vi "Directional Speed Sensors Page.vi"(8 "error in (no error)":errorcluster, 11 "Node Ptr":T1 format="%.0x") -> (0 "error out":errorcluster)   [LabVIEW 2013, in "Engine Simulation Toolkit System Explorer.lvlib"]
uses:
  Engine Simulation Toolkit System Explorer.lvlib
  <vilib>/NI Veristand/Custom Device API/Custom Device Item Ref.ctl
  Shared/Properties.vi
  Shared/Constants and GUIDs.vi
  <vilib>/NI Veristand/Custom Device API/Custom Device API.lvlib
  Shared/Engine Simulation Toolkit Shared.lvlib
  <vilib>/NI Veristand/Custom Device Tools/Custom Device Utility Library/Custom Device Utility Library.lvlib
panel:
  in  "remove":bool
  in  "add":bool
  in  "DirSpeed listbox":i32[](listbox) caption="Available Directional Speed Sensors"
  in  "Header":cluster{"Section Name":string}={"Section Name"="Directional Speed Sensors"}
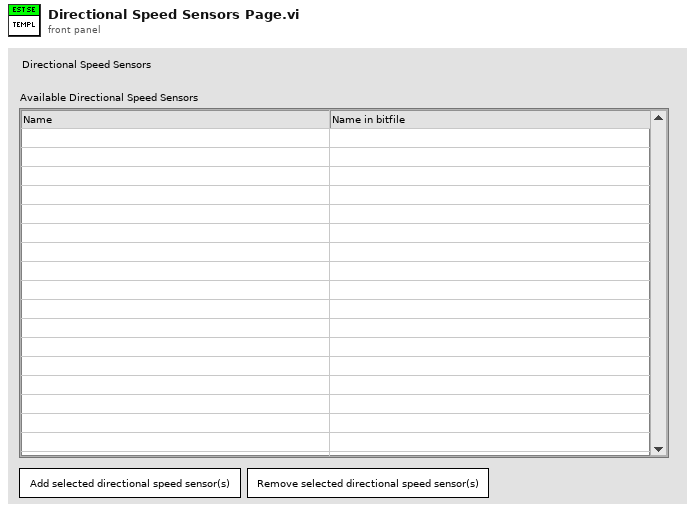
[diagram p1: front panel]
types:
  T1 = typedef "Custom Device API.lvlib/Custom Device Item Ref.ctl" = u64
  T2 = enum8{"Enabled", "Disabled", "Disabled and Grayed Out"}
  T3 = typedef "Custom Device API.lvlib/Custom Device Commands.ctl" = enum16{"Default", "Item renamed", "Shutdown", "Dynamic button pressed"}
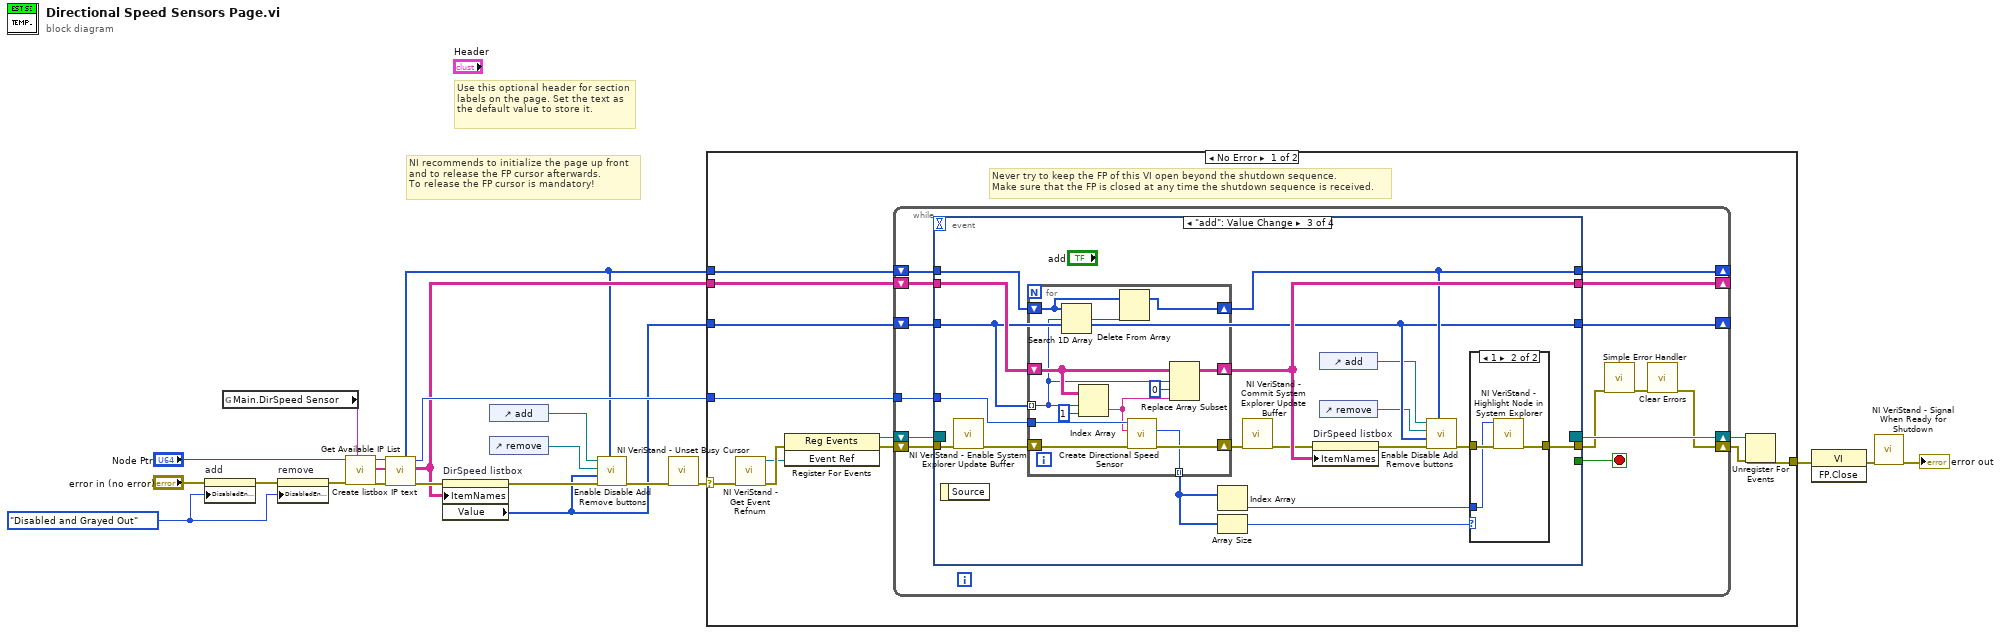
[diagram p0: block diagram]
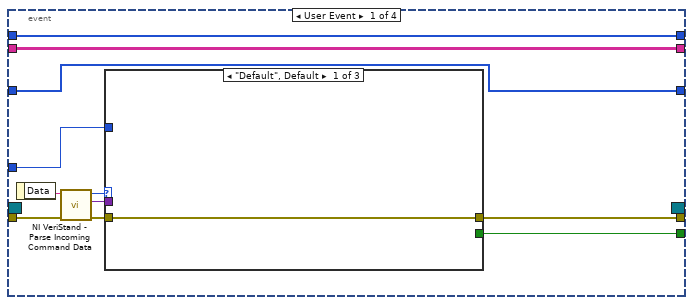
[diagram p2: hidden frame]
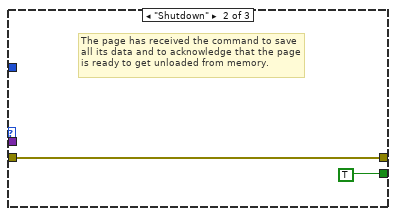
[diagram p3: hidden frame]
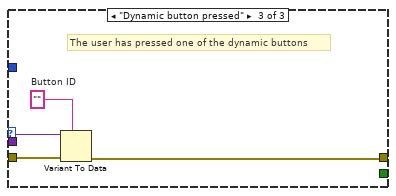
[diagram p4: hidden frame]
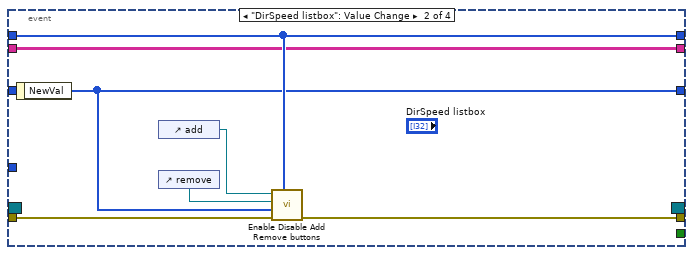
[diagram p5: hidden frame]
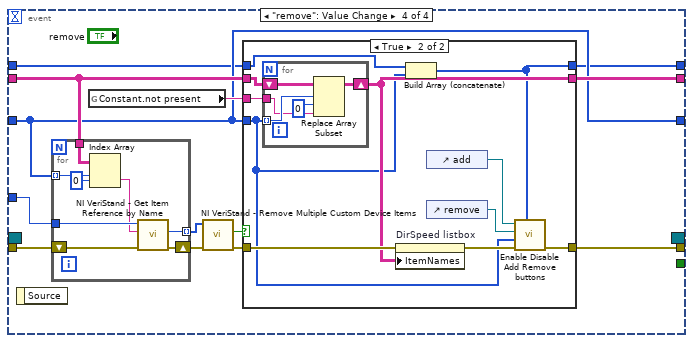
[diagram p7: hidden frame]
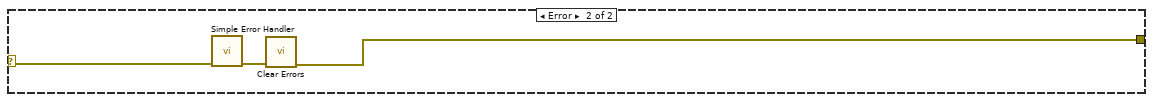
[diagram p9: hidden frame]
diagram:
  w7 = T2."Disabled and Grayed Out" ("Disabled")
  # "Use this optional header for section labels on the page. Set the text as the default value to store it."
  # "NI recommends to initialize the page up front\nand to release the FP cursor afterwards.\nTo release the FP cursor is mandatory!"
  n1 = property on="add" class="Bool"(error in="error in (no error)", "DisabledEnum"=w7) -> (error out=w9:errorcluster)  [unwired: 1 in, 1 out]
  n2 = global read "Properties.vi" "Main.DirSpeed Sensor"() -> (w15:string)
  n3 = property on="remove" class="Bool"(error in=w9, "DisabledEnum"=w7) -> (error out=w8:errorcluster)  [unwired: 1 in, 1 out]
  n4 = call "Get Available IP List.vi"("ip list property name"=w15, "error in (no error)"=w8, "Item Ref in"="Node Ptr") -> ("error out"=w17:errorcluster, "ips available"=w12:string[], "Item Ref out"=w14:T1)  [unwired: 6 in]
  n5 = call "Create listbox IP text.vi"("error in (no error)"=w17, "ips available"=w12, "Section Ref in"=w14) -> ("error out"=w11:errorcluster, "listbox text"=w10:string[][], "Section Ref out"=w13:T1, "not present item indexes"=w2:i32[])  [unwired: 5 in]
  n6 = property on="DirSpeed listbox" class="MCListbox (strict)"(error in=w11, "ItemNames"=w10) -> (error out=w4:errorcluster, "Value"=w1:i32[])  [unwired: 1 in, 1 out]
  n7 = control-ref of="add"() -> (w5:refnum<vi>)
  n8 = control-ref of="remove"() -> (w6:refnum<vi>)
  n9 = call "Enable Disable Add Remove buttons.vi"("not present item indexes"=w2, "error in (no error)"=w4, "selected items"=w1, "remove button"=w6, "add button"=w5) -> ("error out"=w3:errorcluster)  [unwired: 6 in]
  n10 = call <vilib>:"NI VeriStand - Unset Busy Cursor.vi"("error in (no error)"=w3) -> ("error out"=w19:errorcluster)  [unwired: 10 out]
  n11 = case shown="No Error" w19 {
    selector: w19 -> [w26 w151]
    tunnel: [w31 w149] -> w22
    tunnel: w13 -> [w27 _]
    tunnel: w10 -> [w25 _]
    tunnel: w2 -> [w24 _]
    tunnel: w1 -> [w23 _]
    frame No Error {
      # "Never try to keep the FP of this VI open beyond the shutdown sequence.\nMake sure that the FP is closed at any time the shutdown sequence is received."
      n12 = call <vilib>:"NI VeriStand - Get Event Refnum.vi"("error in (no error)"=w26) -> ("error out"=w34:errorcluster, "Event Ref"=w30:refnum<user-event>)  [unwired: 9 out]
      n13 = register-events(error in=w34, w30) -> (reference out=w28:refnum<event-registration>, error out=w29:errorcluster)  [unwired: 1 in]
      n14 = while {
        tunnel: w27 -> [w44]
        shift-right: [w41] -> w32
        shift-left: w29 -> [w47]
        shift-right: [w48] -> w33
        shift-left: w28 -> [w46]
        shift-right: [w38] -> _
        shift-left: w23 -> [w37]
        shift-right: [w35] -> _
        shift-left: w24 -> [w39]
        shift-right: [w36] -> _
        shift-left: w25 -> [w40]
        stop <- w45 stop-if-true
        n15 = event shown="[2] \"add\": Value Change" {
          selector: w46 -> [_ _ _ _]
          dyn-events: [_ _ _ _] -> w48
          timeout: _ -> [_ _ _ _]
          tunnel: w47 -> [w59 w73 w91 w120]
          tunnel: [w55 _ _ _] -> w45
          tunnel: [w54 w72 w76 w121] -> w43
          tunnel: w44 -> [w53 _ w90 w119]
          tunnel: w40 -> [w50 w67 w89 w114]
          tunnel: w39 -> [w49 w69 w88 w110]
          tunnel: [w51 w68 w83 w111] -> w38
          tunnel: w37 -> [w51 _ w83 w111]
          tunnel: [w50 w67 w86 w112] -> w36
          tunnel: [w49 w69 w84 w109] -> w35
          event User Event {
            n16 = event-data() -> ("Data"=w58:string)  [unwired: 1 out]
            n17 = call <vilib>:"NI VeriStand - Parse Incoming Command Data.vi"("error in (no error)"=w59, "Incoming data"=w58) -> ("error out"=w57:errorcluster, "Outgoing data"=w52:variant, "Action"=w56:T3)  [unwired: 7 out]
            n18 = case shown="\"Default\", Default" w56 {
              tunnel: w57 -> [w60 w61 w66]
              tunnel: [_ TRUE _] -> w55
              tunnel: [w60 w61 w63] -> w54
              tunnel: w53 -> [_ _ _]
              tunnel: w52 -> [_ _ w65]
              frame "Default", Default {
              }
              frame "Shutdown" {
                # "The page has received the command to save all its data and to acknowledge that the page is ready to get unloaded from memory."
              }
              frame "Dynamic button pressed" {
                w64 = ""  # Button ID
                # "The user has pressed one of the dynamic buttons"
                n19 = Variant To Data(error in=w66, type=w64, Variant=w65) -> (error out=w63:errorcluster)  [unwired: 1 out]
              }
            }
          }
          event "DirSpeed listbox": Value Change {
            n20 = event-data() -> ("NewVal"=w68:i32[])  [unwired: 1 out]
            n21 = control-ref of="add"() -> (w71:refnum<vi>)
            n22 = control-ref of="remove"() -> (w70:refnum<vi>)
            n23 = call "Enable Disable Add Remove buttons.vi"("not present item indexes"=w69, "error in (no error)"=w73, "selected items"=w68, "remove button"=w70, "add button"=w71) -> ("error out"=w72:errorcluster)  [unwired: 6 in]
          }
          event "add": Value Change {
            n24 = event-data() -> ()  [unwired: 2 out]
            n25 = call <vilib>:"NI VeriStand - Enable System Explorer Update Buffer.vi"("error in (no error)"=w91) -> ("error out"=w79:errorcluster)  [unwired: 10 in]
            n26 = for {
              tunnel: w90 -> [w106]
              shift-right: [w107] -> w87
              shift-left: w79 -> [w108]
              tunnel: w83 -> [w100] mode=indexing
              shift-right: [w103] -> w86
              shift-left: w89 -> [w104]
              shift-right: [w97] -> w84
              shift-left: w88 -> [w99]
              tunnel: [w96] -> w78 mode=indexing
              n27 = Search 1D Array(1D array=w99, element=w100) -> (index of element=w98:i32)  [unwired: 1 in]
              n28 = Index Array(array=w104, index (row)=w100, index (col)=1 ("disabled index (col)")) -> (element=w101:string)
              n29 = Delete From Array(array=w99, index=w98) -> (array with subset deleted=w97:i32[])  [unwired: 1 in, 1 out]
              n30 = call "Create Directional Speed Sensor.vi"("error in (no error)"=w108, "dir speed sensor name"=w101, "Section Ptr"=w106) -> ("error out"=w107:errorcluster, "dir speed sensor ref"=w96:T1)  [unwired: 6 in, 1 out]
              n31 = Replace Array Subset(array=w104, new element=w101, index (row)=w100, index (col)=0 ("disabled index (col)")) -> (w103:string[][])
            }
            n32 = Index Array(array=w78) -> (element=w74:T1)  [unwired: 1 in]
            n33 = Array Size(array=w78) -> (size(s)=w77:i32)
            n34 = call <vilib>:"NI VeriStand - Commit System Explorer Update Buffer.vi"("error in (no error)"=w87) -> ("error out"=w80:errorcluster)  [unwired: 10 in]
            n35 = property on="DirSpeed listbox" class="MCListbox (strict)"(error in=w80, "ItemNames"=w86) -> (error out=w85:errorcluster)  [unwired: 1 in, 1 out]
            n36 = control-ref of="add"() -> (w82:refnum<vi>)
            n37 = control-ref of="remove"() -> (w81:refnum<vi>)
            n38 = call "Enable Disable Add Remove buttons.vi"("not present item indexes"=w84, "error in (no error)"=w85, "selected items"=w83, "remove button"=w81, "add button"=w82) -> ("error out"=w75:errorcluster)  [unwired: 6 in]
            n39 = case shown="1" w77 {
              tunnel: [w92 w94] -> w76
              tunnel: w75 -> [w92 w95]
              tunnel: w74 -> [_ w93]
              frame Default {
              }
              frame 1 {
                n40 = call <vilib>:"NI VeriStand - Highlight Node in System Explorer.vi"("error in (no error)"=w95, "Item Ref in"=w93) -> ("error out"=w94:errorcluster)  [unwired: 8 in, 1 out]
              }
            }
          }
          event "remove": Value Change {
            n41 = event-data() -> ()  [unwired: 2 out]
            n42 = for {
              tunnel: w111 -> [w147] mode=indexing
              tunnel: w114 -> [w148]
              tunnel: w119 -> [w144]
              tunnel: [w141] -> w117 mode=indexing
              shift-right: [w143] -> w118
              shift-left: w120 -> [w145]
              n43 = Index Array(array=w148, index (row)=w147, index (col)=0 ("disabled index (col)")) -> (element=w142:string)
              n44 = call <vilib>:"NI VeriStand - Get Item Reference by Name.vi"("error in (no error)"=w145, "Item Name"=w142, "Parent Ref in"=w144) -> ("error out"=w143:errorcluster, "Item Ref"=w141:T1)  [unwired: 5 in, 2 out]
            }
            n45 = global read "Constants and GUIDs.vi" "Constant.not present"() -> (w113:string)
            n46 = call <vilib>:"NI VeriStand - Remove Multiple Custom Device Items.vi"("error in (no error)"=w118, "Item Refs in"=w117) -> ("error out"=w116:errorcluster, "Deleted?"=w115:bool)  [unwired: 8 in]
            n47 = case shown="True" w115 {
              tunnel: [w123 w134] -> w121
              tunnel: w116 -> [w123 w131]
              tunnel: w111 -> [_ w126]
              tunnel: w114 -> [w124 w130]
              tunnel: w113 -> [_ w129]
              tunnel: [w124 w128] -> w112
              tunnel: w110 -> [w122 w127]
              tunnel: [w122 w125] -> w109
              frame False {
              }
              frame True {
                n48 = for {
                  tunnel: w126 -> [w138] mode=indexing
                  shift-right: [w139] -> w128
                  shift-left: w130 -> [w140]
                  tunnel: w129 -> [w136]
                  n49 = Replace Array Subset(array=w140, new element=w136, index (row)=w138, index (col)=0 ("disabled index (col)")) -> (w139:string[][])
                }
                n50 = property on="DirSpeed listbox" class="MCListbox (strict)"(error in=w131, "ItemNames"=w128) -> (error out=w135:errorcluster)  [unwired: 1 in, 1 out]
                n51 = Build Array (concatenate)(w127, w126) -> (w125:i32[])
                n52 = control-ref of="add"() -> (w133:refnum<vi>)
                n53 = control-ref of="remove"() -> (w132:refnum<vi>)
                n54 = call "Enable Disable Add Remove buttons.vi"("not present item indexes"=w125, "error in (no error)"=w135, "selected items"=w126, "remove button"=w132, "add button"=w133) -> ("error out"=w134:errorcluster)  [unwired: 6 in]
              }
            }
          }
        }
        n55 = call <vilib>:"Simple Error Handler.vi"("error in (no error)"=w43) -> ("error out"=w42:errorcluster)  [unwired: 1 in, 7 out]
        n56 = call <vilib>:"Clear Errors.vi"("error in (no error)"=w42) -> ("error out"=w41:errorcluster)  [unwired: 6 out]
      }
      n57 = Unregister For Events(event registration refnum=w33, error in=w32) -> (error out=w31:errorcluster)
    }
    frame Error {
      n58 = call <vilib>:"Simple Error Handler.vi"("error in (no error)"=w151) -> ("error out"=w150:errorcluster)  [unwired: 1 in, 7 out]
      n59 = call <vilib>:"Clear Errors.vi"("error in (no error)"=w150) -> ("error out"=w149:errorcluster)  [unwired: 6 out]
    }
  }
  n60 = invoke class="VI" method="FP.Close"(error in=w22) -> (error out=w21:errorcluster)  [unwired: 2 in, 2 out]
  n61 = call <vilib>:"NI VeriStand - Signal When Ready for Shutdown.vi"("error in (no error)"=w21) -> ("error out"=→"error out":errorcluster)  [unwired: 10 out]
